vi "Is Class Descendand of Class.vi"(8 "Error In":errorcluster, 10 "Parent ClassName":string, 11 "ClassName":string) -> (0 "Error Out":errorcluster, 3 "is Class descendant?":bool)   [LabVIEW 2018]
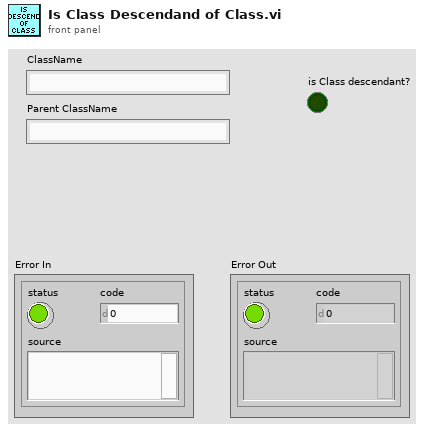
[diagram p1: front panel]
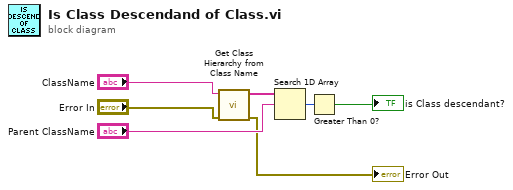
[diagram p0: block diagram]
diagram:
  n1 = call <vilib>:"Get Class Hierarchy from Class Name.vi"("error in (no error)"="Error In", "Class Name"="ClassName") -> ("error out"=→"Error Out":errorcluster, "Class Hierarchy"=w6:string[])  [unwired: 8 in]
  n2 = Search 1D Array(1D array=w6, element="Parent ClassName") -> (index of element=w4:i32)  [unwired: 1 in]
  n3 = Greater Than 0?(x=w4) -> (x > 0?=→"is Class descendant?":bool)
